vi "Save As Commented Sif.vi"(10 "comment":string, 11 "path":string) -> (1 "function return":u32, 2 "comment out":string, 3 "path out":string)   [LabVIEW 2018, in "AndorSDK.lvlib"]
doc: "EXPNETTYPE unsigned int WINAPI SaveAsCommentedSif(char * path, char * comment);"
uses:
  AndorSDK.lvlib
  ATMCD32D.dll
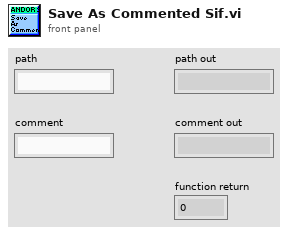
[diagram p1: front panel]
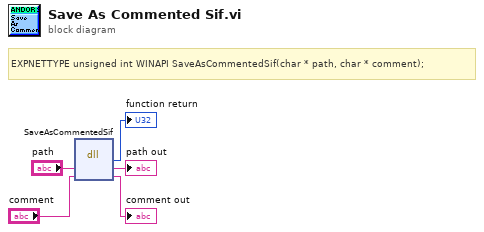
[diagram p0: block diagram]
diagram:
  # "EXPNETTYPE unsigned int WINAPI SaveAsCommentedSif(char * path, char * comment);"
  n1 = dll-call lib="PTH2babs E\nPersönliches02 - Arbeit03-HiwijobsLabviewCodelibANDOR\tAndor SDK\nATMCD32D.*" fn="SaveAsCommentedSif"("path"="path", "comment"="comment") -> (→"function return":u32, "path"=→"path out":string, "comment"=→"comment out":string)  [unwired: 3 in, 2 out]
